vi "Get BD Active.vi"(8 "error in (no error)":errorcluster) -> (0 "error out":errorcluster, 2 "BD Active":bool, 3 "VI Ref":refnum<vi>)   [LabVIEW 2019, in "Window.lvlib"]
doc: "Finds the top-most open block diagram, and returns the corresponding VI reference. If no block diagrams are open, returns an empty reference."
uses:
  Window.lvlib
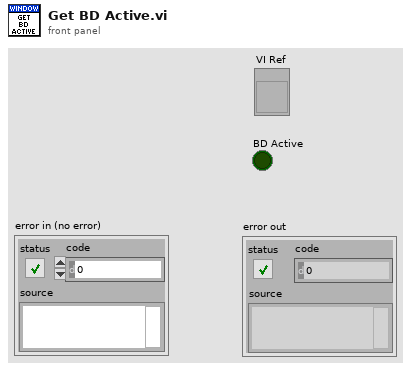
[diagram p1: front panel]
types:
  T1 = enum32{"Invalid", "Standard", "Closed", "Hidden", "Minimized", "Maximized"}
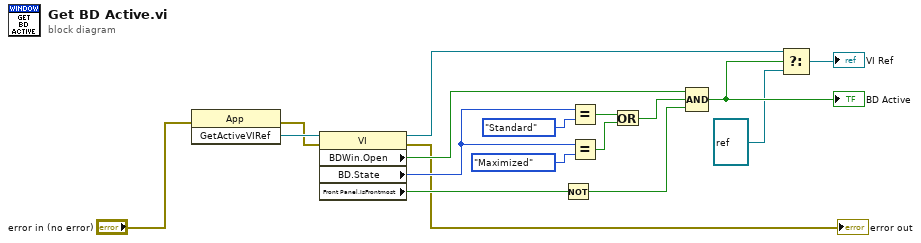
[diagram p0: block diagram]
diagram:
  n1 = invoke class="App" method="GetActiveVIRef"(error in="error in (no error)") -> (error out=w2:errorcluster, "GetActiveVIRef"=w17:refnum<vi>)  [unwired: 2 in, 1 out]
  n2 = property class="VI"(reference=w17, error in=w2) -> (reference out=w7:refnum<vi>, error out=→"error out":errorcluster, "BDWin.Open"=w14:bool, "BD.State"=w12:T1, "Front Panel.IsFrontmost"=w16:bool)
  n3 = Not(x=w16) -> (.not. x?=w13:bool)
  n4 = Equal?(x=w12, y=T1."Standard") -> (x = y?=w10:bool)
  n5 = Equal?(x=w12, y=T1."Maximized") -> (x = y?=w9:bool)
  n6 = Or(x=w10, y=w9) -> (x .or. y?=w8:bool)
  n7 = Compound Arithmetic op=AND(w14, w8, w13) -> (w6:bool)
  "BD Active" <- w6
  n8 = Select(t=w7, s=w6, f=refnum<vi> refnum) -> (s? t:f=→"VI Ref":refnum<vi>)
